vi "Python String to LabVIEW Data (String).vi"(8 "error in (no error)":errorcluster, 9 "type (String)":string, 10 "Python String":string) -> (0 "error out":errorcluster, 2 "LabVIEW Data":string)   [LabVIEW 2020, in "jki_python_data_tools.lvlib"]
doc: "Reads a value associated with key in a specified section of the configuration data identified by refnum. If \"key\" input is not specified, the name of the variant object is used as the key. the \"found?\" output will be TRUE for compount objects (clusters) only if all elements (recursively) are found.\n\nFor example a Boolean named \"Enable\" with a value of TRUE would correspond to the key-value pair:\n\nEnable=TRUE"
uses:
  jki_python_data_tools.lvlib
panel:
  # "Copyright © 2003-2009 JKI. All rights reserved.\n\nAuthor:\nPhilippe Guerit [philippe.guerit@jameskring.com]\nJim Kring [jim.kring@jameskring.com]\n\nThis library is provided \"AS IS\" ,WITHOUT WARRANTIES OR \nCONDITIONS OF ANY KIND, either express or implied.\n\nJames Kring, Inc. -- http://www.jameskring.com"
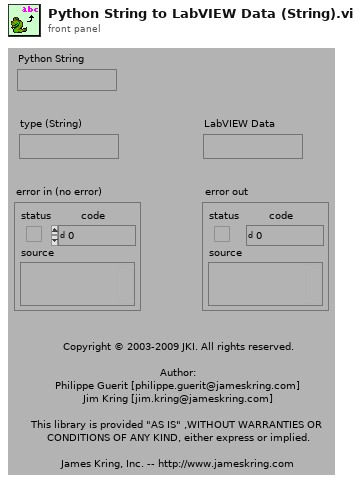
[diagram p1: front panel]
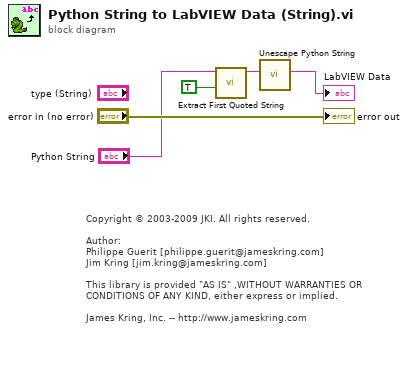
[diagram p0: block diagram]
diagram:
  # "Copyright © 2003-2009 JKI. All rights reserved.\n\nAuthor:\nPhilippe Guerit [philippe.guerit@jameskring.com]\nJim Kring [jim.kring@jameskring.com]\n\nThis library is provided \"AS IS\" ,WITHOUT WARRANTIES OR \nCONDITIONS OF ANY KIND, either express or implied.\n\nJames Kring, Inc. -- http://www.jameskring.com"
  n1 = call "Extract First Quoted String.vi"("Strip Quotes (FALSE)"=TRUE, "Quoted String"="Python String") -> ("First Quoted String"=w3:string)  [unwired: 7 in, 2 out]
  n2 = call "Unescape Python String.vi"("Escaped Python String"=w3) -> ("Unescaped String"=→"LabVIEW Data":string)  [unwired: 10 in]
  "error out" <- "error in (no error)"
